vi "updater.vi"() -> ()   [LabVIEW 2020]
uses:
  <vilib>/Utility/error.llb/DialogType.ctl
panel:
  out "String":string
  in  "SHUT DOWN":bool
  in  "UPDATE":bool
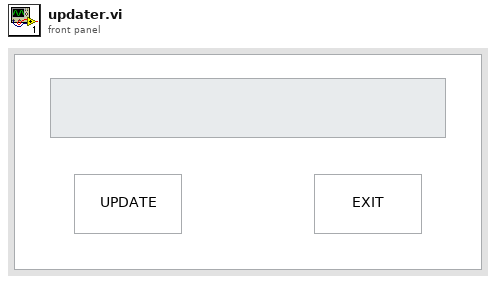
[diagram p1: front panel]
types:
  T1 = typedef "DialogType.ctl" = u16
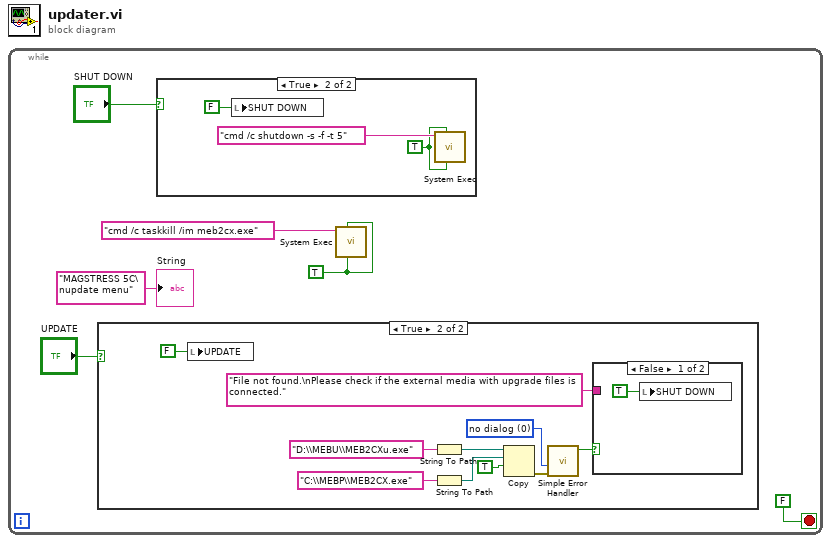
[diagram p0: block diagram]
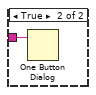
[diagram p4: hidden frame]
diagram:
  n1 = while {
    stop <- FALSE stop-if-true
    w2 = TRUE ("wait until completion? (T)")
    n2 = case shown="True" "UPDATE" {
      frame False {
      }
      frame True {
        w15 = T1 0 items=["no dialog", "OK message", "continue or stop message", "OK message + warnings", "continue/stop + warnings"] ("type of dialog (OK msg:1)")
        n3 = local write "UPDATE"(FALSE ("UPDATE")) -> ()
        n4 = String To Path(string="D:\\MEBU\\MEB2CXu.exe") -> (path=w11:path)
        n5 = String To Path(string="C:\\MEBP\\MEB2CX.exe") -> (path=w12:path)
        n6 = Copy(9:TRUE ("overwrite (F)"), 10:w12, 11:w11) -> (0:w10:errorcluster)  [unwired: 2 in, 2 out]
        n7 = call <vilib>:"Simple Error Handler.vi"("type of dialog (OK msg:1)"=w15, "error in (no error)"=w10) -> ("error?"=w19:bool)  [unwired: 3 in, 4 out]
        n8 = case shown="False" w19 {
          tunnel: "File not found.\nPlease check if the external media with upgrade files is connected." -> [_ w21]
          frame False {
            n9 = local write "SHUT DOWN"(TRUE ("UPDATE")) -> ()
          }
          frame True {
            n10 = One Button Dialog(message=w21) -> ()  [unwired: 1 in, 1 out]
          }
        }
      }
    }
    n11 = case shown="True" "SHUT DOWN" {
      frame False {
      }
      frame True {
        w8 = TRUE ("wait until completion? (T)")
        n12 = local write "SHUT DOWN"(FALSE ("SHUT DOWN")) -> ()
        n13 = call <vilib>:"System Exec.vi"("run minimized? (F)"=w8, "wait until completion? (T)"=w8, "command line"="cmd /c shutdown -s -f -t 5") -> ()  [unwired: 5 in, 4 out]
      }
    }
    n14 = call <vilib>:"System Exec.vi"("run minimized? (F)"=w2, "wait until completion? (T)"=w2, "command line"="cmd /c taskkill /im meb2cx.exe") -> ()  [unwired: 5 in, 4 out]
    "String" <- "MAGSTRESS 5C\nupdate menu" ("String")
  }
